vi "22w XY.vi"(0 "picture":picture caption="图片", 1 "desired font(Application)":T5(ring)=enum."Application Font" caption="所需字体（应用程序）", 3 "[user-specified font]":T6 caption="[用户定义字体]", 5 "data":cluster{"x":dbl, "y":dbl}[](array[cluster]) caption="数据" {"y" format="%0.2f"; "x" format="%0.2f"}, 7 "dimensions (w,h)":cluster{"width":i16, "height":i16} caption="尺寸（宽度、高度）", 11 "top left point(0, 0)":cluster{"x":i16, "y":i16} caption="左上角点(0, 0)", 12 "cartesian axis attributes":T7={"x minimum"=0.0, "x maximum"=0.0, "x log?"=FALSE, "x precision"=1, "x format"=enum."Decimal", "y minimum"=0.0, "y maximum"=0.0, "y log?"=FALSE, "y precision"=1, "y format"=enum."Decimal"} caption="直角坐标属性" {"x minimum" format="%0.2f"; "x maximum" format="%0.2f"; "y minimum" format="%0.2f"; "y maximum" format="%0.2f"}, 13 "cartesian grid cosmetics":T4={"line color"=6710886, "text color"=13421772, "tick length(3)"=3, "crossing axes"=FALSE, "visible grid?"=TRUE} caption="直角网格修饰", 14 "XY plot cosmetics":T3={"plot color"=16776960, "XY plot type"=enum."connected points", "baseline"=0.0} caption="XY曲线修饰" {"baseline" format="%0.2f"}, 15 "[sized scatter plot cosmetics]":T1={"min size"=1, "max size"=5, "maps to max size"=5, "color array"=[16776960, 65280, 16711680, 255]} caption="[带大小的分散图修饰]") -> (4 "new picture":picture caption="新图片")   [LabVIEW 2020]
doc: "获取图片和点数组，添加显示数据的XY图的图片。"
uses:
  <vilib>/picture/cartesn2.llb/XY Plot Type.ctl
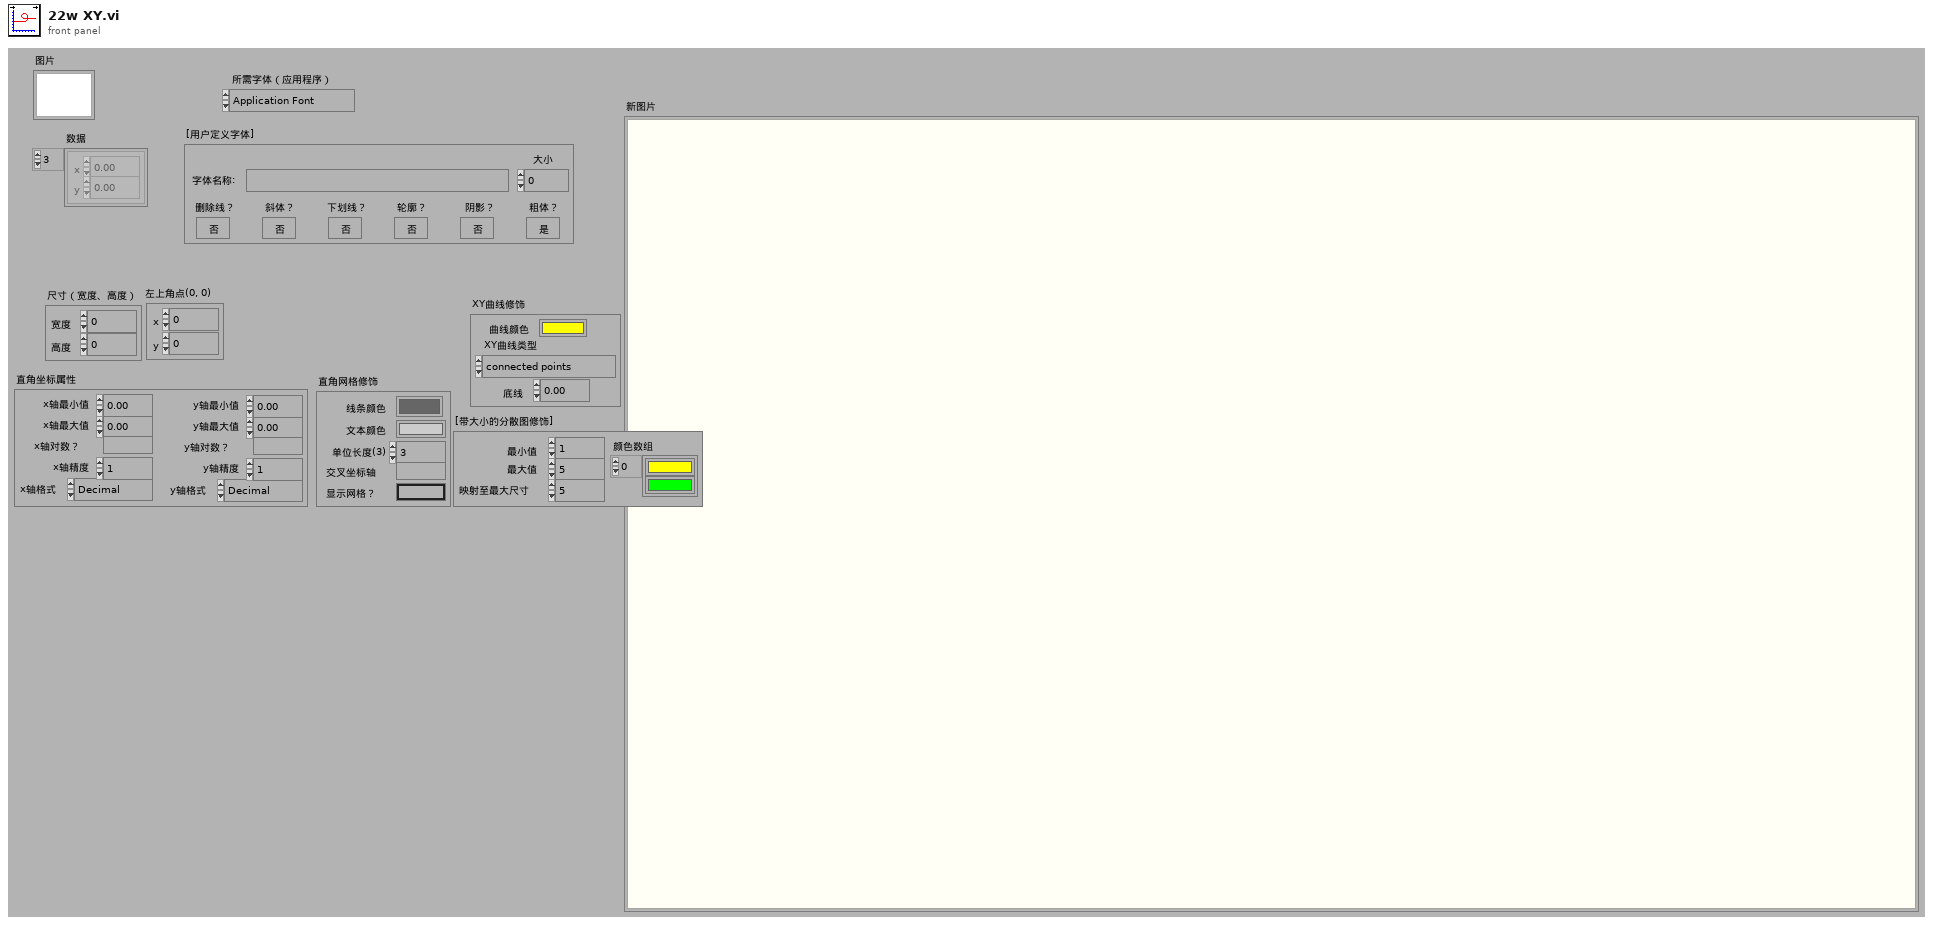
[diagram p1: front panel]
types:
  T1 = cluster{"min size":i16, "max size":i16, "maps to max size":i16, "color array":u32[]}
  T2 = typedef "XY Plot Type.ctl" = enum16{"points", "squares", "circles", "connected points", "connected squares", "connected circles", "comb plot", "sized scatter plot", "sized-colored scatter plot", "min-max lines"}
  T3 = cluster{"plot color":u32, "XY plot type":T2, "baseline":dbl}
  T4 = cluster{"line color":u32, "text color":u32, "tick length(3)":i16, "crossing axes":bool, "visible grid?":bool}
  T5 = enum16{"User-specified Font", "Application Font", "System Font", "Dialog Font"}
  T6 = cluster{"Font Name:":string, "Size":i16, "Strikeout?":bool, "Italic?":bool, "Underline?":bool, "Outline?":bool, "Shadow?":bool, "Bold?":bool}
  T7 = cluster{"x minimum":dbl, "x maximum":dbl, "x log?":bool, "x precision":u8, "x format":enum8{"Decimal", "Scientific", "Engineering", "Binary", "Octal", "Hex"}, "y minimum":dbl, "y maximum":dbl, "y log?":bool, "y precision":u8, "y format":enum8{"Decimal", "Scientific", "Engineering", "Binary", "Octal", "Hex"}}
  T8 = cluster{"left":i16, "top":i16, "right":i16, "bottom":i16}
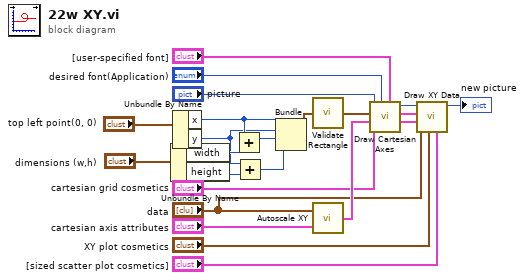
[diagram p0: block diagram]
diagram:
  n1 = Unbundle By Name("dimensions (w,h)") -> ("width"=w9:i16, "height"=w8:i16)
  n2 = Unbundle By Name("top left point(0, 0)") -> ("x"=w7:i16, "y"=w6:i16)
  n3 = Add(x=w7, y=w9) -> (x+y=w5:i16)
  n4 = Add(x=w6, y=w8) -> (x+y=w4:i16)
  n5 = Bundle("x"=w7, "y"=w6, w5, w4) -> (w3:cluster{"x":i16, "y":i16, i16, i16})  [unwired: 1 in]
  n6 = call <vilib>:"Validate Rectangle.vi"("rect"=w3) -> ("valid rect"=w21:T8)
  n7 = call <vilib>:"Autoscale XY.vi"("axis attributes"="cartesian axis attributes", "xy data"="data") -> ("axis attributes"=w22:T7)
  n8 = call <vilib>:"Draw Cartesian Axes.vi"("[user-specified font]"="[user-specified font]", "desired font(Application)"="desired font(Application)", "grid cosmetics"="cartesian grid cosmetics", "axis attributes"=w22, "bounding rect"=w21, "picture"="picture") -> ("y scale factors"=w17:cluster{"a":dbl, "b":dbl, "log?":bool}, "x scale factors"=w16:cluster{"a":dbl, "b":dbl, "log?":bool}, "new picture"=w14:picture)  [unwired: 3 in]
  n9 = call <vilib>:"Draw XY Data.vi"("[sized scatter plot cosmetics]"="[sized scatter plot cosmetics]", "xy cosmetics"="XY plot cosmetics", "xy data"="data", "y scale factors"=w17, "x scale factors"=w16, "picture"=w14) -> ("new picture"=→"new picture":picture)  [unwired: 5 in]
